vi "h.ACQ.GetStreamingSensors.vi"(8 "error in":errorcluster, 10 "Timeout":i32=10000, 11 "Connection ID In":refnum<k5>) -> (0 "error out":errorcluster, 2 "Sensor Data":T1, 3 "Connection ID Out":refnum<k5>)   [LabVIEW 2016, in "h.Library.lvlib"]
doc: "This vi retrieves data from a streaming data socket.\n\n<b>Connection ID In</b> - is a network connection refnum that uniquely identifies the TCP connection\n<b>Timeout</b> - specifies the maximum amount of time, in milliseconds, for the function to complete\n<b>error in</b> - describes error conditions that occur before this node runs. This input provides standard error functionality\n<b>Connection ID Out</b> - returns the same value as connection ID\n<b>Peaks Data</b> - peaks wvl data\n<b>error out</b> - contains error information. This output provides standard error out functionality."
uses:
  h.Library.lvlib
  COMM/CTL/h.COMM.Command Status Enum.ctl
  CTL/h.ACQ.SensorData.ctl
panel:
  out "Status":T2
  # "Hyperion Get Streaming Sensors"
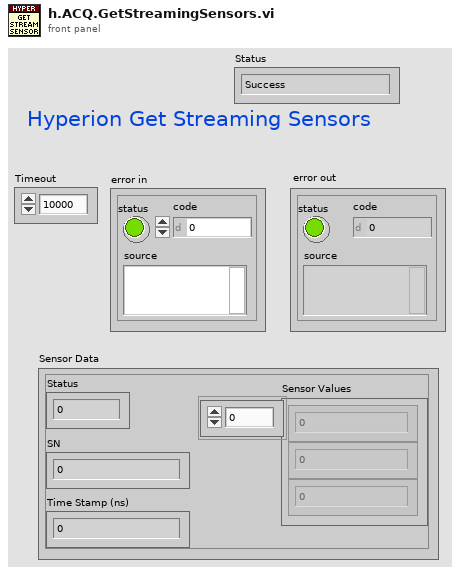
[diagram p1: front panel]
types:
  T1 = typedef "h.Library.lvlib/h.ACQ.SensorData.ctl" = cluster{"SN":u64, "Time Stamp (ns)":u64, "Status":u16, "Sensor Values":dbl[]}
  T2 = typedef "h.Library.lvlib/h.COMM.Command Status Enum.ctl" = enum8{"Success", "Failed", "Error", "AccessDenied", "InvalidCommand", "InvalidNumberArguments", "InvalidArgument", ""}
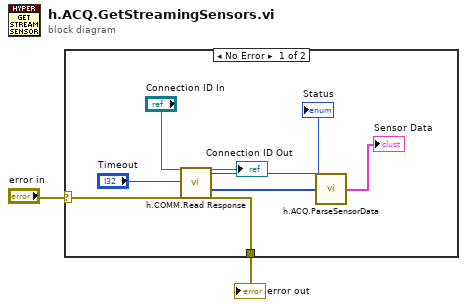
[diagram p0: block diagram]
diagram:
  n1 = case shown="No Error" "error in" {
    selector: "error in" -> [w7 w11]
    tunnel: [w10 w11] -> w1
    frame No Error {
      n2 = call "h.COMM.Read Response.vi"("Connection ID"="Connection ID In", "Timeout"="Timeout", "error in"=w7) -> ("Connection ID"=→"Connection ID Out":refnum<k5>, "Status"=→"Status":T2, "Content"=w5:u8[], "error out"=w10:errorcluster)  [unwired: 17 in, 4 out]
      n3 = call "h.ACQ.ParseSensorData.vi"("Raw Sensor Data"=w5) -> ("Sensor Data"=→"Sensor Data":T1)
    }
    frame Error {
    }
  }
  "error out" <- w1
